vi "ExposeLogInfo.vi"(10 "Action time [ms]":dbl=-1.0, 11 "message":string) -> ()   [LabVIEW 2017]
uses:
  Core/ExposeGlobals.vi
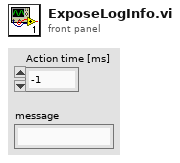
[diagram p1: front panel]
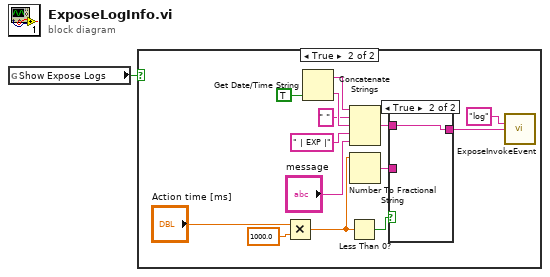
[diagram p0: block diagram]
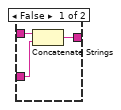
[diagram p3: hidden frame]
diagram:
  n1 = global read "ExposeGlobals.vi" "Show Expose Logs"() -> (w1:bool)
  n2 = case shown="True" w1 {
    frame False {
    }
    frame True {
      n3 = Multiply(x="Action time [ms]", y=1000.0) -> (x*y=w7:dbl)
      n4 = Get Date/Time String(want seconds? (F)=TRUE) -> (date string=w10:string, time string=w12:string)  [unwired: 2 in]
      n5 = Less Than 0?(x=w7) -> (x < 0?=w3:bool)
      n6 = Concatenate Strings(w10, " " ("string"), w12, " | EXP |" ("string"), "message") -> (w6:string)
      n7 = Number To Fractional String(number=w7) -> (F-format string=w5:string)  [unwired: 3 in]
      n8 = case shown="True" w3 {
        tunnel: w6 -> [w18 w19]
        tunnel: w5 -> [w17 _]
        tunnel: [w16 w19] -> w4
        frame False {
          n9 = Concatenate Strings(w18, w17) -> (w16:string)
        }
        frame True {
        }
      }
      n10 = call "ExposeInvokeEvent.vi"("name"="log", "Data"=w4) -> ()  [unwired: 13 in, 1 out]
    }
  }
